vi "LED Initialization.vi"(8 "Device ID":dbl=-1.0, 11 "CANifier Name":string) -> ()   [LabVIEW 2019]
uses:
  Globals/LED_Globals.vi
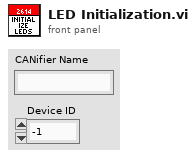
[diagram p1: front panel]
types:
  T1 = typedef "CTRE_CANifier_DeviceRef.ctl" = cluster{"DeviceStatus":errorcluster, "Device Number":u8, "Handle":u64, "UsageFrame":u32, "Library Path":path}
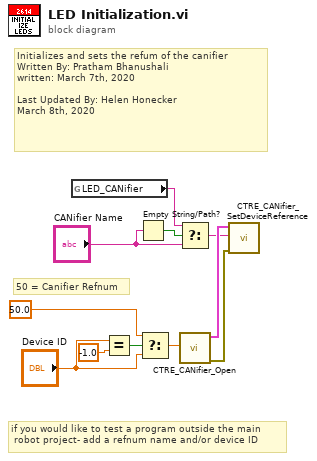
[diagram p0: block diagram]
diagram:
  # "if you would like to test a program outside the main\n robot project- add a refnum name and/or device ID"
  # "50 = Canifier Refnum"
  # "Initializes and sets the refum of the canifier\nWritten By: Pratham Bhanushali\nwritten: March 7th, 2020\n\nLast Updated By: Helen Honecker\nMarch 8th, 2020"
  n1 = global read "LED_Globals.vi" "LED_CANifier"() -> (w3:string)
  n2 = Equal?(x="Device ID", y=-1.0) -> (x = y?=w8:bool)
  n3 = Empty String/Path?(string/path="CANifier Name") -> (empty?=w4:bool)
  n4 = Select(t=50.0, s=w8, f="Device ID") -> (s? t:f=w5:dbl)
  n5 = Select(t=w3, s=w4, f="CANifier Name") -> (s? t:f=w1:string)
  n6 = call <vilib>:"CTRE_CANifier_Open.vi"("Device Number"=w5) -> ("error out"=w11:errorcluster, "CANifierDevRef"=w10:T1)  [unwired: 9 in]
  n7 = call <vilib>:"CTRE_CANifier_SetDeviceReference.vi"("error in (no error)"=w11, "refnum name"=w1, "CANifierDevRef"=w10) -> ()  [unwired: 7 in, 2 out]
